vi "HXGetTerm.vi"(1 "stateInfoUSIConnect out":T1) -> (0 "BlockNodeState.Terminal Data":T16[](array[typedef]) {"Terminal Flags" format="%.0b"})   [LabVIEW 2017]
uses:
  <vilib>/BlockNodeSupport/TerminalData.ctl
  <vilib>/Platform/storage/lvStorage.llb/_stateInfoWriteProps.ctl
  <vilib>/Platform/storage/lvStorage.llb/dataStorageParams.ctl
  <vilib>/Platform/storage/lvStorage.llb/_selectedProp.ctl
  <vilib>/Platform/storage/lvStorage.llb/dataModel.ctl
  <vilib>/Platform/storage/Storage.llb/usiTypeDef.ctl
  <vilib>/Platform/storage/Storage.llb/usiPropDef.ctl
  <vilib>/express/express shared/ex_EditUserDefinedProperties/usiDataType.ctl
  <vilib>/Platform/storage/Storage.llb/specialProperties.ctl
  <vilib>/Platform/storage/Storage.llb/usiOverwriteOptions.ctl
  <vilib>/Platform/storage/lvStorage.llb/TerminalDef.ctl
  <vilib>/Platform/storage/lvStorage.llb/_TerminalStyle.ctl
  <vilib>/Utility/XNodeSupport.llb/XRect32.ctl
  <vilib>/Platform/storage/Storage.llb/usiSequenceRepresentation.ctl
  <vilib>/Platform/storage/lvStorage.llb/channelType.ctl
  <vilib>/Platform/storage/lvStorage.llb/_dataTerminals.ctl
  <vilib>/Platform/storage/lvStorage.llb/_stringsToBeTranslated.ctl
  <vilib>/XNodeSupport/NI_XNodeSupport.lvlib
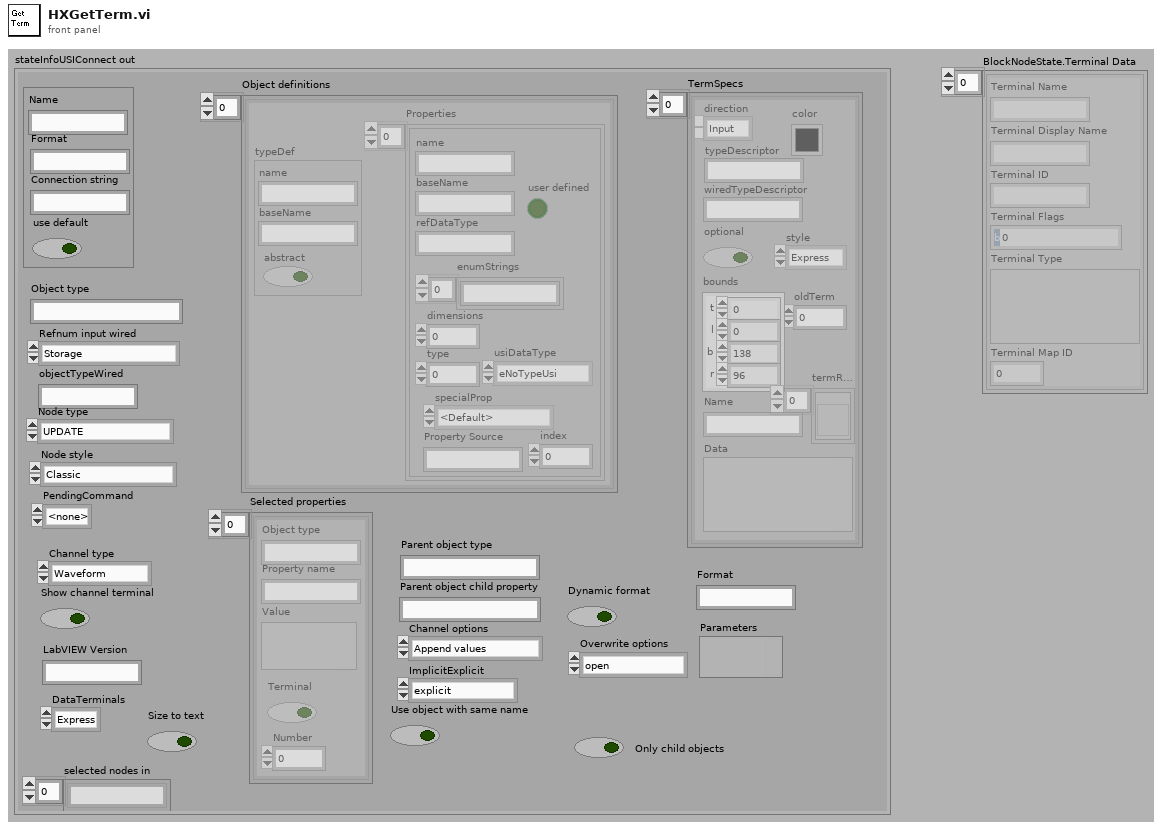
[diagram p1: front panel]
types:
  T1 = typedef "_stateInfoWriteProps.ctl" = cluster{"Data storage parameters":T2, "Object type":string, "Selected properties":T3[], "Object definitions":T4[], "Refnum input wired":enum16{"Storage", "Generic object", "Typed object", "<none>"}, "Parent object type":string, "Parent object child property":string, "Channel options":T9, "PendingCommand":enum16{"<none>", "SelPopUp", "Init"}, "Node style":enum16{"Classic", "Express"}, "Only child objects":bool, "TermSpecs":T10[], "objectTypeWired":string, "Dynamic format":bool, "Overwrite options":enum16{"open", "open or create", "create or replace", "create", "open (read only)"}, "Parameters":variant, "Format":string, "Node type":enum16{"UPDATE", "READ", "QUERY", "CREATE CHILD", "CREATE", "CONNECT", "DISCONNECT"}, "ImplicitExplicit":T13, "Channel type":T14, "Use object with same name":bool, "Show channel terminal":bool, "LabVIEW Version":string, "DataTerminals":T15, "Size to text":bool, "selected nodes in":string[]}
  T2 = typedef "dataStorageParams.ctl" = cluster{"Name":string, "Format":string, "Connection string":string, "use default":bool}
  T3 = typedef "_selectedProp.ctl" = cluster{"Object type":string, "Property name":string, "Value":variant, "Terminal":bool, "Number":i32}
  T4 = typedef "dataModel.ctl" = cluster{"typeDef":T5, "Properties":T6[]}
  T5 = typedef "usiTypeDef.ctl" = cluster{"name":string, "baseName":string, "abstract":bool}
  T6 = typedef "usiPropDef.ctl" = cluster{"name":string, "baseName":string, "refDataType":string, "dimensions":i32, "type":i32, "user defined":bool, "enumStrings":string[], "usiDataType":T7, "specialProp":T8, "Property Source":string, "index":i32}
  T7 = typedef "usiDataType.ctl" = enum16{"eNoTypeUsi", "eInt8Usi", "eInt16Usi", "eInt32Usi", "eInt64Usi", "eUInt8Usi", "eUInt16Usi", "eUInt32Usi", "eUInt64Usi", "eFloat32Usi", "eFloat64Usi", "- 0", "- 1", "- 2", "- 3", "- 4", "- 5", "- 6", "- 7", "- 8", "- 9", "eString8Usi", "eString16Usi", "eStringUsi", "eEnumUsi", "- 10", "- 11", "- 12", "- 13", "- 14", "eTimeUsi", "- 15", "- 16", "- 17", "- 18", "- 19", "- 20", "- 21", "- 22", "- 23", "eInstanceUsi", "eStoreUsi"}
  T8 = typedef "specialProperties.ctl" = enum16{"<Default>", "Channel Values", "AppendReplace", "ChannelFlags", "ValueFlags", "ImplicitExplicit", "InsertIndex", "ValuesCount", "ComparisonOperator", "Cluster", "DAQmx Channel"}
  T9 = typedef "usiOverwriteOptions.ctl" = enum16{"Append values", "Replace values at index", "Replace all values", "Append if timeline aligns"}
  T10 = typedef "TerminalDef.ctl" = cluster{"direction":enum16{"Input", "Output"}, "typeDescriptor":string, "color":u32, "oldTerm":i32, "style":T11, "optional":bool, "bounds":T12, "termRefs":refnum<vi>[], "Name":string, "Data":variant, "wiredTypeDescriptor":string}
  T11 = typedef "_TerminalStyle.ctl" = enum16{"Express", "Collapsed", "Internal"}
  T12 = typedef "XRect32.ctl" = cluster{"t":i32, "l":i32, "b":i32, "r":i32}
  T13 = typedef "usiSequenceRepresentation.ctl" = enum16{"explicit", "implicit"}
  T14 = typedef "channelType.ctl" = enum16{"Waveform", "Array of Double", "Array of String", "DDT", "Array of UInt8", "Array of Int16", "Array of Int32", "Array of Single", "Array of DateTime", "Array of Waveform", "none", "DateTime", "String", "Double", "Single", "UInt8", "Int16", "Int32"}
  T15 = typedef "_dataTerminals.ctl" = enum16{"Express", "Cluster"}
  T16 = typedef "TerminalData.ctl" = cluster{"Terminal Name":string, "Terminal Display Name":string, "Terminal ID":string, "Terminal Flags":i32, "Terminal Type":variant, "Terminal Map ID":i32}
  T17 = enum16{"UPDATE", "READ", "QUERY", "CREATE CHILD", "CREATE", "CONNECT", "DISCONNECT"}
  T18 = typedef "_stringsToBeTranslated.ctl" = enum16{"Properties", "View as icon", "query all data", "Load Storage VI parameters into memory", "Dynamically assign format", "Enumerated type", "Time stamp", "Configure", "Size to text", "Untitled", "storage refnum", "Load waveform data", "TDM (...)", "LVM (...)", "CSV (...)", "DYN (...)", "WrittenByLabVIEW", "TDMS", "out"}
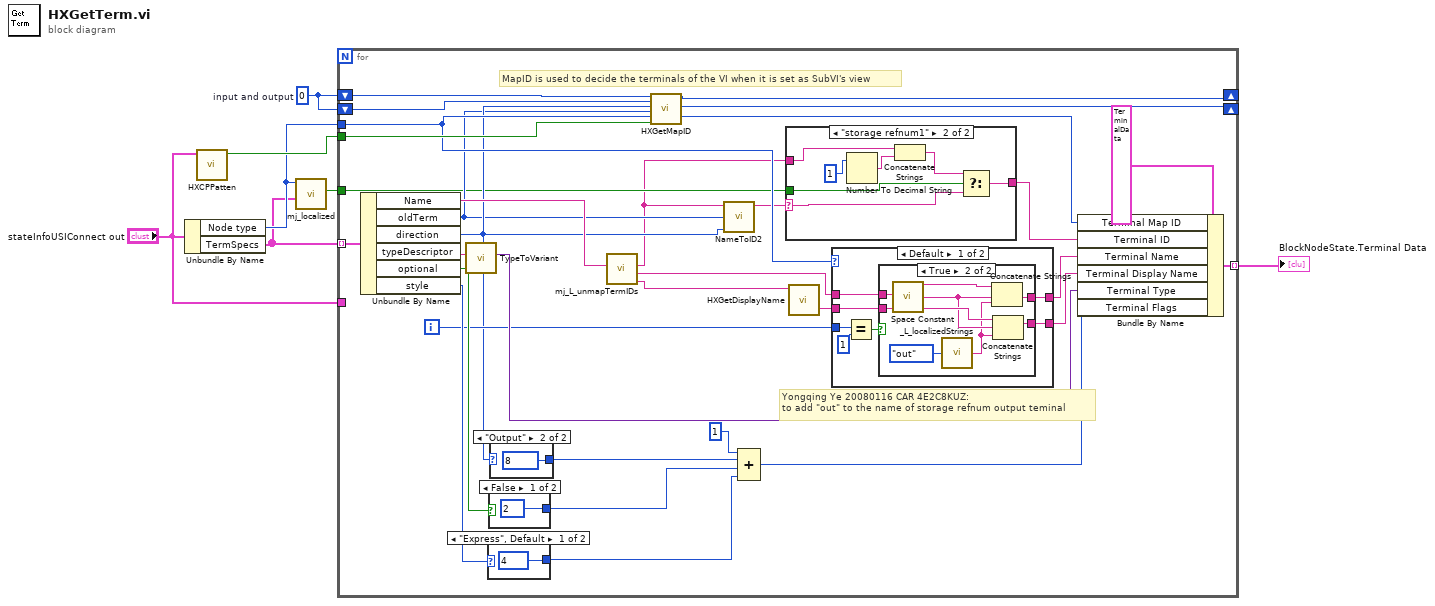
[diagram p0: block diagram]
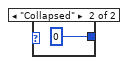
[diagram p5: hidden frame]
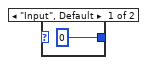
[diagram p6: hidden frame]
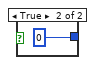
[diagram p7: hidden frame]
diagram:
  w7 = 0  # input and output
  n1 = Unbundle By Name("stateInfoUSIConnect out") -> ("Node type"=w3:T17, "TermSpecs"=w2:T10[])
  n2 = call <vilib>:"HXCPPatten.vi"("stateInfo"="stateInfoUSIConnect out") -> ("x .or. y?"=w6:bool)  [unwired: 10 out]
  n3 = call <vilib>:"mj_localized.vi"("TermSpecs"=w2, "Node type"=w3) -> ("improperly localized?"=w1:bool)  [unwired: 9 in]
  n4 = for {
    tunnel: w2 -> [w39] mode=indexing
    shift-right: [w31] -> _
    shift-left: w7 -> [w33]
    shift-right: [w30] -> _
    shift-left: w7 -> [w32]
    tunnel: w6 -> [w28]
    tunnel: w3 -> [w21]
    tunnel: [w22] -> w5 mode=indexing
    tunnel: "stateInfoUSIConnect out" -> [_]
    tunnel: w1 -> [w9]
    i -> [w19]
    # "Yongqing Ye 20080116 CAR 4E2C8KUZ:\nto add \"out\" to the name of storage refnum output teminal"
    # "MapID is used to decide the terminals of the VI when it is set as SubVI's view"
    n5 = Unbundle By Name(w39) -> ("Name"=w17:string, "oldTerm"=w11:i32, "direction"=w12:enum16{"Input", "Output"}, "typeDescriptor"=w37:string, "optional"=w35:bool, "style"=w34:T11)
    n6 = call <vilib>:"TypeToVariant.vi"("typeCode"=w37) -> ("Variant"=w36:variant)  [unwired: 1 in, 5 out]
    n7 = case shown="\"Express\", Default" w34 {
      tunnel: [4 0] -> w25
      frame "Express", Default {
      }
      frame "Collapsed" {
      }
    }
    n8 = case shown="False" w35 {
      tunnel: [2 0] -> w26
      frame False {
      }
      frame True {
      }
    }
    n9 = case shown="\"Output\"" w12 {
      tunnel: [0 8] -> w27
      frame "Input", Default {
      }
      frame "Output" {
      }
    }
    n10 = call <vilib>:"mj_L_unmapTermIDs.vi"("DNL_Name"=w17) -> ("DNL_DisplayName"=w15:string, "DNL_LocalizedTermName"=w18:string, "DNL_TermID"=w8:string)  [unwired: 1 in, 5 out]
    n11 = call <vilib>:"HXGetMapID.vi"("input"=w33, "output"=w32, "direction"=w12, "OldTerm"=w11, "Node type"=w21, "Boolean"=w28) -> ("Input"=w31:i32, "Output"=w30:i32, "MapID"=w29:i32)  [unwired: 11 out]
    n12 = call <vilib>:"NameToID2.vi"("direction"=w12, "old term"=w11, "name"=w8) -> ("String Out"=w10:string)  [unwired: 8 out]
    n13 = Compound Arithmetic op=ADD(1, w27, w26, w25) -> (w23:i32)
    n14 = case shown="\"storage refnum1\"" w10 {
      selector: w10 -> [w40 w42]
      tunnel: [w40 w44] -> w13
      tunnel: w9 -> [_ w45]
      tunnel: w8 -> [_ w41]
      frame Default {
      }
      frame "storage refnum1" {
        n15 = Number To Decimal String(number=i16 1 ("width (-)")) -> (decimal integer string=w47:string)  [unwired: 1 out]
        n16 = Concatenate Strings(w41, w47) -> (w43:string)
        n17 = Select(t=w43, s=w45, f=w42) -> (s? t:f=w44:string)
      }
    }
    n18 = call <vilib>:"HXGetDisplayName.vi"("String"=w15) -> ("String 2"=w20:string)  [unwired: 10 out]
    n19 = case shown="Default" w21 {
      tunnel: w18 -> [w51 w65]
      tunnel: w20 -> [w50 w64]
      tunnel: w19 -> [w54 _]
      tunnel: [w49 w65] -> w16
      tunnel: [w48 w64] -> w14
      frame Default {
        n20 = Equal?(x=w54, y=1) -> (x = y?=w52:bool)
        n21 = case shown="True" w52 {
          tunnel: w51 -> [w56 w59]
          tunnel: w50 -> [w55 w63]
          tunnel: [w56 w62] -> w49
          tunnel: [w55 w61] -> w48
          frame False {
          }
          frame True {
            n22 = call <vilib>:"Space Constant.vi"() -> ("String"=w58:string)
            n23 = call <vilib>:"_L_localizedStrings.vi"(1:_stringsToBeTranslated."out") -> (0:w57:string)
            n24 = Concatenate Strings(w59, w58, w57) -> (w62:string)
            n25 = Concatenate Strings(w63, w58, w57) -> (w61:string)
          }
        }
      }
      frame "CONNECT", "DISCONNECT" {
      }
    }
    n26 = Bundle By Name(cluster=T16 {"Terminal Name"="", "Terminal Display Name"="", "Terminal ID"="", "Terminal Flags"=0, "Terminal Type"=variant, "Terminal Map ID"=0} ("XNTerminalData"), "Terminal Map ID"=w29, "Terminal ID"=w13, "Terminal Name"=w16, "Terminal Display Name"=w14, "Terminal Type"=w36, "Terminal Flags"=w23) -> (w22:T16)
  }
  "BlockNodeState.Terminal Data" <- w5
